vi "calculate_offset_and_range.vi"(8 "error in (no error)":errorcluster, 11 "Image in":refnum<class "Image.lvclass">) -> (0 "error out":errorcluster, 1 "range":dbl, 2 "offset / minimum":dbl, 3 "Image out":refnum<class "Image.lvclass">, 4 "maximum":dbl)   [LabVIEW 2010, in "Image.lvclass"]
uses:
  Image.lvclass
  storage_mode.ctl
  error_codes_ring.ctl
  ErrorController/ErrorController/class_data.vi
  ErrorController/ErrorController/ErrorController.lvclass
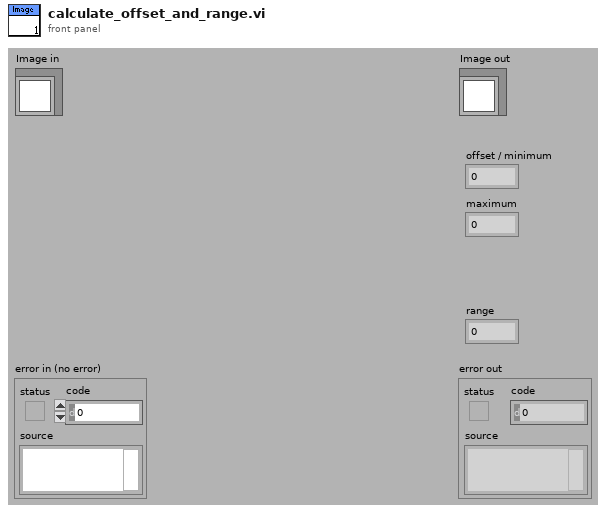
[diagram p1: front panel]
types:
  T1 = typedef "Image.lvclass/storage_mode.ctl" = enum16{"RAM", "disk"}
  T2 = typedef "Image Type" = u32
  T3 = typedef "Image.lvclass/error_codes_ring.ctl" = u16
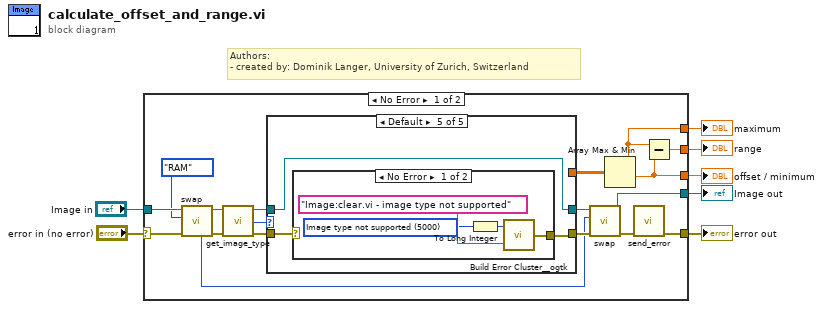
[diagram p0: block diagram]
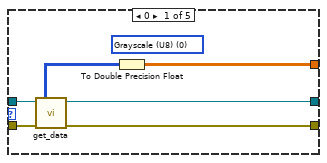
[diagram p2: hidden frame]
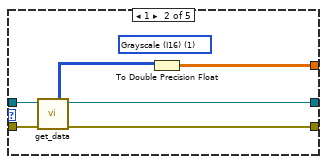
[diagram p3: hidden frame]
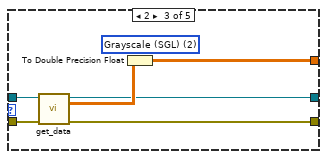
[diagram p4: hidden frame]
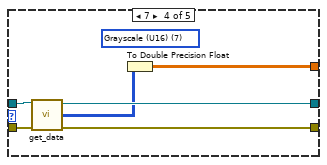
[diagram p5: hidden frame]
diagram:
  # "Authors: \n- created by: Dominik Langer, University of Zurich, Switzerland"
  n1 = case shown="No Error" "error in (no error)" {
    selector: "error in (no error)" -> [w19 w59]
    tunnel: [w8 w59] -> w6
    tunnel: [w13 w58] -> w4
    tunnel: "Image in" -> [w17 w58]
    tunnel: [w24 _] -> w3
    tunnel: [w23 _] -> w2
    tunnel: [w22 _] -> w1
    frame No Error {
      n2 = call-dynamic "swap.vi"("error in (no error)"=w19, "storage type target"=storage_mode."RAM", "Image in"=w17) -> ("error out"=w18:errorcluster, "Image out"=w11:refnum<class "Image.lvclass">, "previous storage mode"=w12:T1)  [unwired: 6 out]
      n3 = call-dynamic "get_image_type.vi"("error in (no error)"=w18, "Image.lvclass in"=w11) -> ("error out"=w10:errorcluster, "Image Type"=w21:T2, "Image.lvclass out"=w20:refnum<class "Image.lvclass">)  [unwired: 7 out]
      n4 = case shown="Default" w21 {
        tunnel: [w26 w32 w39 w47 w51] -> w15
        tunnel: [w31 w34 w40 w45 _] -> w25
        tunnel: w20 -> [w28 w36 w42 w48 w50]
        tunnel: [w27 w33 w38 w46 w50] -> w14
        tunnel: w10 -> [w30 w37 w43 w49 w52]
        frame 0 {
          (unwired) T2 0 items=["Grayscale (U8)", "Grayscale (I16)", "Grayscale (SGL)", "Complex (CSG)", "RGB (U32)", "HSL (U32)", "RGB (U64)", "Grayscale (U16)"] ("Image Type")
          n5 = call-dynamic "get_data.vi"("Image in"=w28, "error in (no error)"=w30) -> ("Image Pixels (U8)"=w29:u8[][], "Image out"=w27:refnum<class "Image.lvclass">, "error out"=w26:errorcluster)  [unwired: 11 out]
          n6 = To Double Precision Float(number=w29) -> (double precision float=w31:dbl[][])
        }
        frame 1 {
          (unwired) T2 1 items=["Grayscale (U8)", "Grayscale (I16)", "Grayscale (SGL)", "Complex (CSG)", "RGB (U32)", "HSL (U32)", "RGB (U64)", "Grayscale (U16)"] ("Image Type")
          n7 = call-dynamic "get_data.vi"("Image in"=w36, "error in (no error)"=w37) -> ("Image Pixels (I16)"=w35:i16[][], "Image out"=w33:refnum<class "Image.lvclass">, "error out"=w32:errorcluster)  [unwired: 11 out]
          n8 = To Double Precision Float(number=w35) -> (double precision float=w34:dbl[][])
        }
        frame 2 {
          (unwired) T2 2 items=["Grayscale (U8)", "Grayscale (I16)", "Grayscale (SGL)", "Complex (CSG)", "RGB (U32)", "HSL (U32)", "RGB (U64)", "Grayscale (U16)"] ("Image Type")
          n9 = call-dynamic "get_data.vi"("Image in"=w42, "error in (no error)"=w43) -> ("Image out"=w38:refnum<class "Image.lvclass">, "Image Pixels (Float)"=w41:sgl[][], "error out"=w39:errorcluster)  [unwired: 11 out]
          n10 = To Double Precision Float(number=w41) -> (double precision float=w40:dbl[][])
        }
        frame 7 {
          (unwired) T2 7 items=["Grayscale (U8)", "Grayscale (I16)", "Grayscale (SGL)", "Complex (CSG)", "RGB (U32)", "HSL (U32)", "RGB (U64)", "Grayscale (U16)"] ("Image Type")
          n11 = call-dynamic "get_data.vi"("Image in"=w48, "error in (no error)"=w49) -> ("Image out"=w46:refnum<class "Image.lvclass">, "Image Pixels (U16)"=w44:u16[][], "error out"=w47:errorcluster)  [unwired: 11 out]
          n12 = To Double Precision Float(number=w44) -> (double precision float=w45:dbl[][])
        }
        frame Default {
          n13 = case shown="No Error" w52 {
            selector: w52 -> [_ w57]
            tunnel: [w56 w57] -> w51
            frame No Error {
              w54 = T3 5000 items=["Image type not supported"=5000] ("Ring")
              n14 = To Long Integer(number=w54) -> (32bit integer=w53:i32)
              n15 = call <userlib>:"Build Error Cluster__ogtk.vi"("String to Prepend to source (\"\")"="Image:clear.vi - image type not supported" ("String to Prepend to source (\"\")"), "code"=w53) -> ("error out"=w56:errorcluster)
            }
            frame Error {
            }
          }
        }
      }
      n16 = call-dynamic "swap.vi"("error in (no error)"=w15, "storage type target"=w12, "Image in"=w14) -> ("error out"=w9:errorcluster, "Image out"=w13:refnum<class "Image.lvclass">)  [unwired: 7 out]
      n17 = Array Max & Min(array=w25) -> (max value=w24:dbl, min value=w23:dbl)  [unwired: 2 out]
      n18 = call "send_error.vi"("error in (no error)"=w9) -> ("error out"=w8:errorcluster)  [unwired: 10 in]
      n19 = Subtract(x=w24, y=w23) -> (x-y=w22:dbl)
    }
    frame Error {
    }
  }
  "error out" <- w6
  "Image out" <- w4
  "offset / minimum" <- w2
  "maximum" <- w3
  "range" <- w1
